vi "PCSMain.Free PHELIX Oscilloscope Instances.vi"(1 "DB Entries":cluster{"Object Name":string, "Class":string}[](array[cluster])) -> (0 "Free Oscilloscope Instances":cluster{"Object Name":string, "Class":string}[](array[cluster]))   [LabVIEW 2014, in "PCSMain.lvlib"]
doc: "This VI gives out all entries which are belonging to the classes PH_BackreflectionMeas, PH_TKDS30xx, PH_Tektronix_7000, and PH_Synchrolock_Watch. This VI is meant to be used in MainGUIs."
uses:
  PCSMain.lvlib
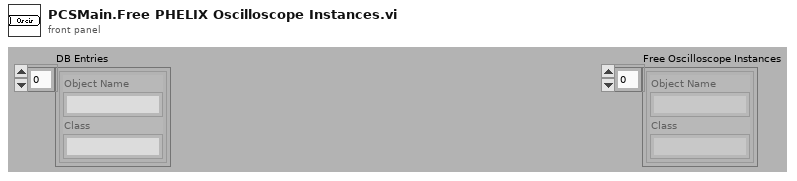
[diagram p1: front panel]
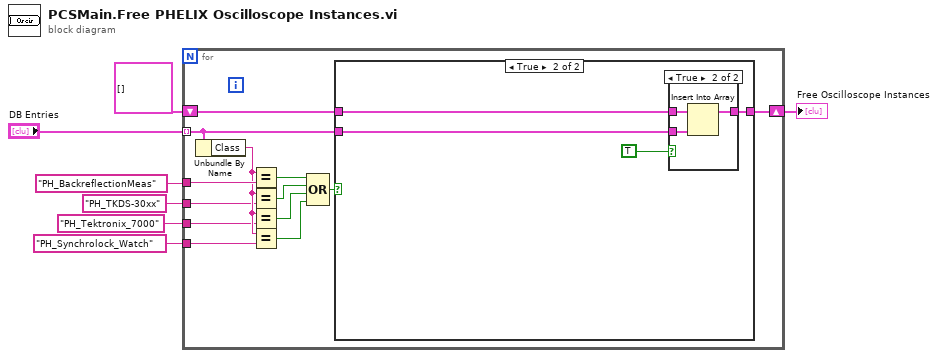
[diagram p0: block diagram]
diagram:
  n1 = for {
    tunnel: "PH_BackreflectionMeas" ("Class") -> [w20]
    tunnel: "DB Entries" -> [w19] mode=indexing
    shift-right: [w18] -> w4
    shift-left: cluster{"Object Name":string, "Class":string}[] [] -> [w17]
    tunnel: "PH_TKDS-30xx" ("Class") -> [w11]
    tunnel: "PH_Tektronix_7000" ("Class") -> [w10]
    tunnel: "PH_Synchrolock_Watch" ("Class") -> [w9]
    n2 = Unbundle By Name(w19) -> ("Class"=w12:string)
    n3 = Equal?(x=w12, y=w20) -> (x = y?=w16:bool)
    n4 = Equal?(x=w12, y=w11) -> (x = y?=w14:bool)
    n5 = Equal?(x=w12, y=w10) -> (x = y?=w13:bool)
    n6 = Equal?(x=w12, y=w9) -> (x = y?=w8:bool)
    n7 = Compound Arithmetic op=OR(w16, w14, w13, w8) -> (w15:bool)
    n8 = case shown="True" w15 {
      tunnel: w19 -> [_ w23]
      tunnel: [w21 w25] -> w18
      tunnel: w17 -> [w21 w24]
      frame False {
      }
      frame True {
        n9 = case shown="True" TRUE {
          tunnel: w23 -> [_ w29]
          tunnel: [w26 w28] -> w25
          tunnel: w24 -> [w26 w27]
          frame False {
          }
          frame True {
            n10 = Insert Into Array(array=w27, new element=w29) -> (w28:cluster{"Object Name":string, "Class":string}[])  [unwired: 1 in]
          }
        }
      }
    }
  }
  "Free Oscilloscope Instances" <- w4
